vi "DB_Ruta_UDL.vi"() -> (3 "UDL ruta":path)   [LabVIEW 2018]
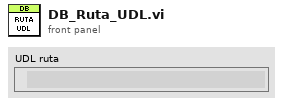
[diagram p1: front panel]
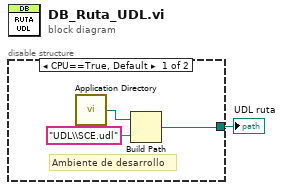
[diagram p0: block diagram]
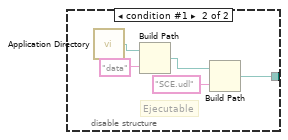
[diagram p2: hidden frame]
diagram:
  n1 = disable-structure shown="CPU==True, Default" {
    disable-tunnel: [w2 w5] -> w1
    frame condition #0 (active) {
      # "Ambiente de desarrollo"
      n2 = call <vilib>:"Application Directory.vi"() -> ("Application Directory"=w3:path)
      n3 = Build Path(base path=w3, name or relative path="UDL\\SCE.udl") -> (appended path=w2:path)
    }
    frame condition #1 {
      # "Ejecutable"
      n4 = call <vilib>:"Application Directory.vi"() -> ("Application Directory"=w9:path)
      n5 = Build Path(base path=w9, name or relative path="data") -> (appended path=w6:path)
      n6 = Build Path(base path=w6, name or relative path="SCE.udl") -> (appended path=w5:path)
    }
  }
  "UDL ruta" <- w1
